vi "Draw Text with Subscripts.vi"(4 "BG color(transparent)":u32, 5 "Autoscale Font Size?":bool, 6 "picture":picture, 7 "Font":T1, 8 "String":string, 9 "alignment(left, top)":T3, 10 "text color(black)":u32, 11 "Draw Area Size":T2) -> (3 "new picture":picture)   [LabVIEW 2012, in "String XControl.xctl"]
uses:
  String XControl.xctl
  <vilib>/Utility/miscctls.llb/LVBoundsTypeDef.ctl
panel:
  out "Font Out":T1
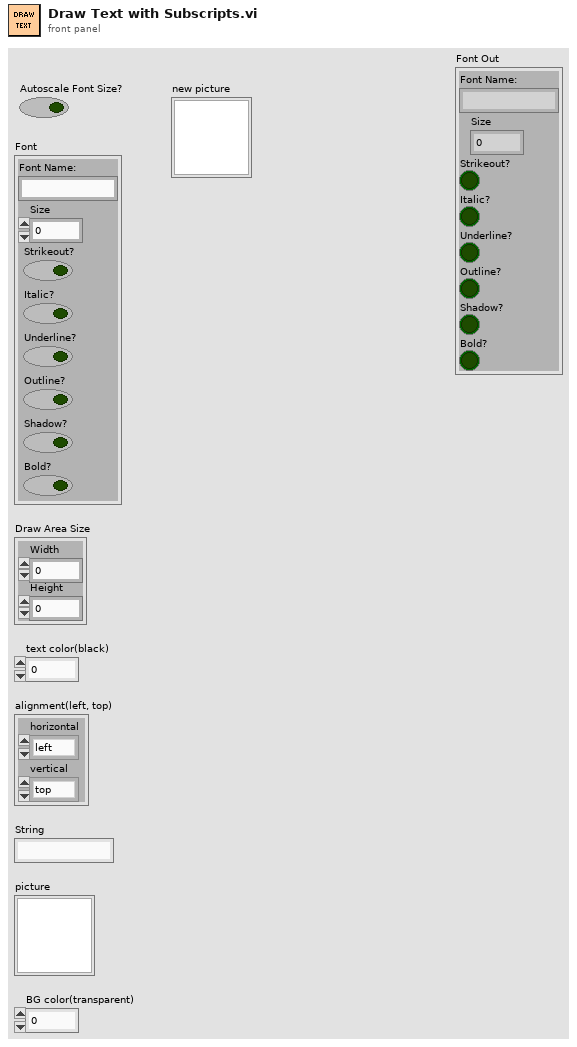
[diagram p1: front panel]
types:
  T1 = cluster{"Font Name:":string, "Size":i16, "Strikeout?":bool, "Italic?":bool, "Underline?":bool, "Outline?":bool, "Shadow?":bool, "Bold?":bool}
  T2 = typedef "LVBoundsTypeDef.ctl" = cluster{"Width":u32, "Height":u32}
  T3 = cluster{"horizontal":enum16{"left", "center", "right"}, "vertical":enum16{"top", "center", "bottom"}}
  T4 = enum16{"User-specified Font", "Application Font", "System Font", "Dialog Font"}
  T5 = cluster{"left":i16, "top":i16, "right":i16, "bottom":i16}
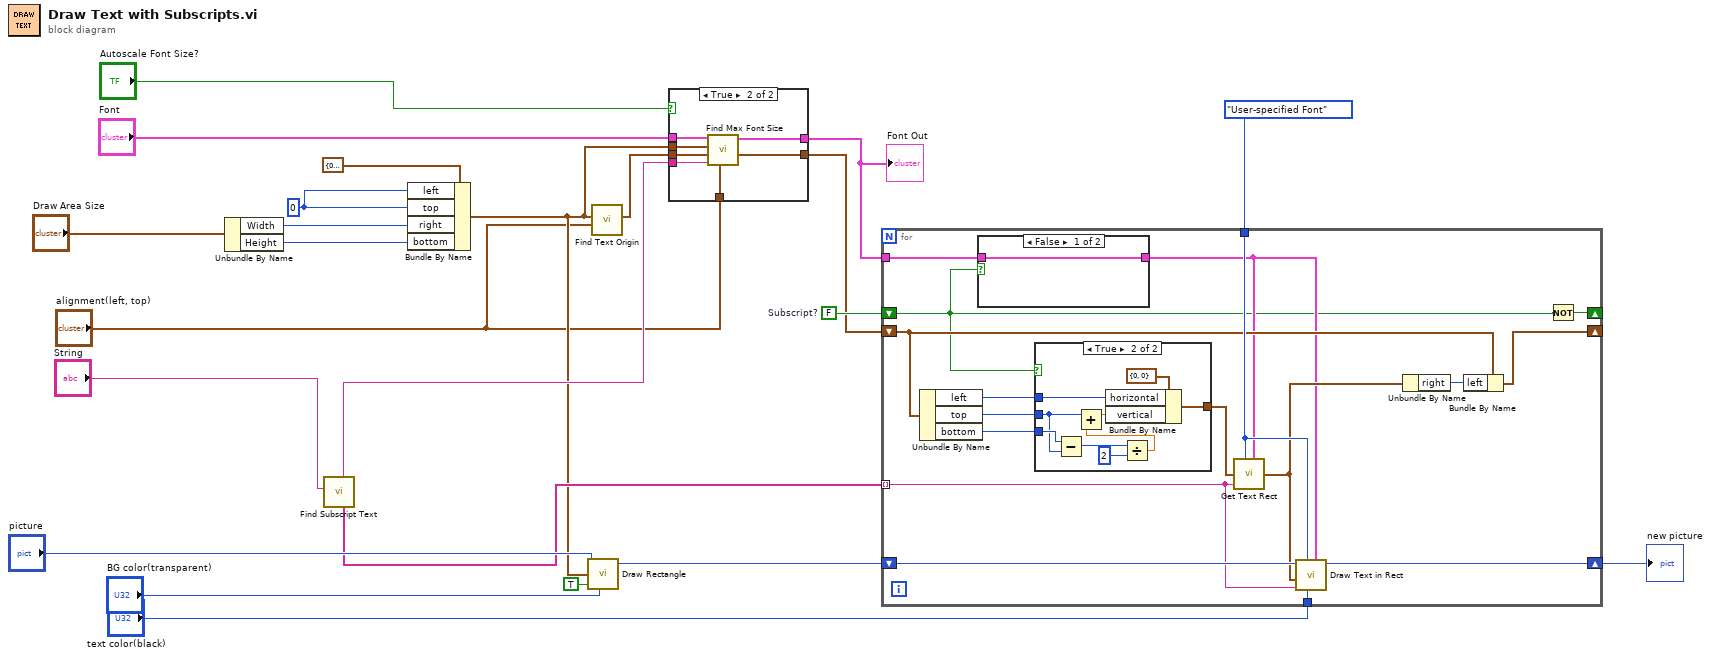
[diagram p0: block diagram]
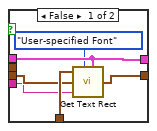
[diagram p2: hidden frame]
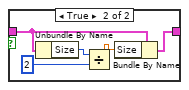
[diagram p3: hidden frame]
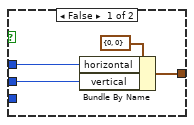
[diagram p4: hidden frame]
diagram:
  w21 = FALSE  # Subscript?
  w5 = i16 0 ("top")
  n1 = Unbundle By Name("Draw Area Size") -> ("Width"=w4:u32, "Height"=w3:u32)
  n2 = call "Find Subscript Text.vi"("String"="String") -> ("interleaved array"=w20:string[], "concatenated string"=w19:string)  [unwired: 7 in, 2 out]
  n3 = Bundle By Name(cluster=T5 {"left"=0, "top"=0, "right"=0, "bottom"=0} ("rect"), "left"=w5, "top"=w5, "right"=w4, "bottom"=w3) -> (w15:T5)
  n4 = call <vilib>:"Draw Rectangle.vi"("picture"="picture", "rect"=w15, "fill?(F)"=TRUE, "color(black)"="BG color(transparent)") -> ("new picture"=w7:picture)  [unwired: 5 in]
  n5 = call "Find Text Origin.vi"("alignment(left, top)"="alignment(left, top)", "Bounding Rectangle"=w15) -> ("origin(0,0)"=w12:cluster{"horizontal":i16, "vertical":i16})  [unwired: 9 in]
  n6 = case shown="True" "Autoscale Font Size?" {
    tunnel: "Font" -> [w28 w36]
    tunnel: w12 -> [w25 w35]
    tunnel: "alignment(left, top)" -> [w29 w34]
    tunnel: [w28 w33] -> w14
    tunnel: w15 -> [_ w32]
    tunnel: [w27 w31] -> w16
    tunnel: w19 -> [w24 w30]
    frame False {
      n7 = call <vilib>:"Get Text Rect.vi"("alignment(left, top)"=w29, "desired font(Application)"=T4."User-specified Font", "origin(0,0)"=w25, "text"=w24, "[user-specified font]"=w28) -> ("rect"=w27:T5)  [unwired: 4 in]
    }
    frame True {
      n8 = call "Find Max Font Size.vi"("alignment(left, top)"=w34, "String"=w30, "Text origin(0,0)"=w35, "Bounding Rect"=w32, "Font In"=w36) -> ("Text Bounding Rect"=w31:T5, "Font Out"=w33:T1)  [unwired: 5 in]
    }
  }
  "Font Out" <- w14
  n9 = for {
    tunnel: T4."User-specified Font" ("desired font(Application)") -> [w47]
    tunnel: "text color(black)" -> [w51]
    tunnel: w14 -> [w40]
    shift-right: [w52] -> w8
    shift-left: w7 -> [w53]
    tunnel: w20 -> [w46] mode=indexing
    shift-right: [w42] -> _
    shift-left: w16 -> [w44]
    shift-right: [w38] -> _
    shift-left: w21 -> [w37]
    n10 = Unbundle By Name(w44) -> ("left"=w50:i16, "top"=w49:i16, "bottom"=w41:i16)
    n11 = case shown="False" w37 {
      tunnel: w40 -> [w54 w59]
      tunnel: [w54 w58] -> w39
      frame False {
      }
      frame True {
        n12 = Unbundle By Name(w59) -> ("Size"=w57:i16)
        n13 = Divide(x=w57, y=i16 2) -> (x/y=w56:dbl)
        n14 = Bundle By Name(cluster=w59, "Size"=w56) -> (w58:T1)
      }
    }
    n15 = case shown="True" w37 {
      tunnel: w50 -> [w62 w71]
      tunnel: w49 -> [w61 w67]
      tunnel: [w60 w70] -> w48
      tunnel: w41 -> [_ w68]
      frame False {
        n16 = Bundle By Name(cluster=cluster{"horizontal":i16, "vertical":i16} {"horizontal"=0, "vertical"=0} ("origin(0,0)"), "horizontal"=w62, "vertical"=w61) -> (w60:cluster{"horizontal":i16, "vertical":i16})
      }
      frame True {
        n17 = Subtract(x=w68, y=w67) -> (x-y=w66:i16)
        n18 = Divide(x=w66, y=i16 2) -> (x/y=w64:dbl)
        n19 = Add(x=w67, y=w64) -> (x+y=w69:dbl)
        n20 = Bundle By Name(cluster=cluster{"horizontal":i16, "vertical":i16} {"horizontal"=0, "vertical"=0} ("origin(0,0)"), "horizontal"=w71, "vertical"=w69) -> (w70:cluster{"horizontal":i16, "vertical":i16})
      }
    }
    n21 = call <vilib>:"Get Text Rect.vi"("desired font(Application)"=w47, "origin(0,0)"=w48, "text"=w46, "[user-specified font]"=w39) -> ("rect"=w45:T5)  [unwired: 5 in]
    n22 = call <vilib>:"Draw Text in Rect.vi"("[user-specified font]"=w39, "text color(black)"=w51, "desired font(Application)"=w47, "text"=w46, "rect"=w45, "picture"=w53) -> ("new picture"=w52:picture)  [unwired: 5 in]
    n23 = Unbundle By Name(w45) -> ("right"=w43:i16)
    n24 = Bundle By Name(cluster=w44, "left"=w43) -> (w42:T5)
    n25 = Not(x=w37) -> (.not. x?=w38:bool)
  }
  "new picture" <- w8
